vi "stringToUTF8ArrayWithLength.vi"(7 "string":string) -> (8 "UTF8[]":u8[](array[numeric]))   [LabVIEW 2013]
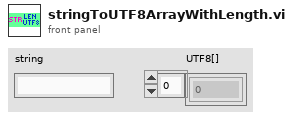
[diagram p1: front panel]
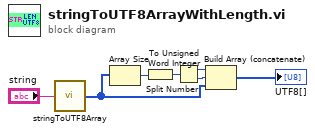
[diagram p0: block diagram]
diagram:
  n1 = call "stringToUTF8Array.vi"("string"="string") -> ("UTF8[]"=w1:u8[])  [unwired: 14 in]
  n2 = Array Size(array=w1) -> (size(s)=w6:i32)
  n3 = To Unsigned Word Integer(number=w6) -> (unsigned 16bit integer=w3:u16)
  n4 = Split Number(x=w3) -> (hi(x)=w4:u8, lo(x)=w5:u8)
  n5 = Build Array (concatenate)(w4, w5, w1) -> (→"UTF8[]":u8[])
